vi "readFlowRateSpec.vi"(1 "Flow range Index":T2 caption="Flow range" items=["0-10 sccm", "0-100 sccm", "0-1000 sccm"], 2 "Channel Index":T1=3 caption="Channel" items=["Channel 1", "Channel 2", "Channel 3", "Channel 4", "Channel 5", "Channel 6", "Channel 7", "Channel 8", "Channel 9", "Channel 10", "Channel 11", "Channel 12", "Channel 13", "Channel 14", "Channel 15", "Channel 16"]) -> (0 "Flow Rate (sccm)":dbl)   [LabVIEW 2011]
uses:
  MFC_Spec.ctl
  AD_Spec.ctl
panel:
  out "Voltage":dbl
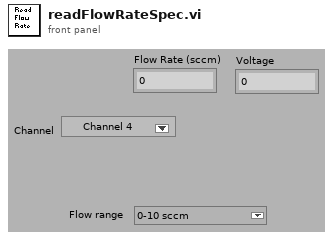
[diagram p1: front panel]
types:
  T1 = typedef "AD_Spec.ctl" = u16
  T2 = typedef "MFC_Spec.ctl" = u16
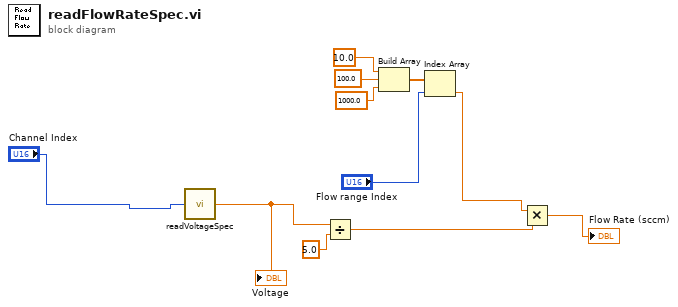
[diagram p0: block diagram]
diagram:
  n1 = call "readVoltageSpec.vi"("Channel"="Channel Index") -> ("Voltage"=w10:dbl)
  "Voltage" <- w10
  n2 = Divide(x=w10, y=5.0) -> (x/y=w9:dbl)
  n3 = Build Array(10.0 ("element"), 100.0 ("element"), 1000.0 ("element")) -> (w8:dbl[])
  n4 = Index Array(array=w8, index="Flow range Index") -> (element=w3:dbl)
  n5 = Multiply(x=w3, y=w9) -> (x*y=→"Flow Rate (sccm)":dbl)
